vi "Teleop.vi"(10 "Match Info":T1={"Autonomous Elapsed Seconds"=0.0, "TeleOp Elapsed Seconds"=0.0, "Disabled Elapsed Seconds"=0.0, "Visited Autonomous"=FALSE, "Visited TeleOp"=FALSE, "Visited Disabled"=FALSE, "Autonomous Settings"={"Autonomous Style"=enum."Independent", "VI Refnum"=refnum}}, 11 "Call Context":T2) -> ()   [LabVIEW 2019]
doc: "This VI is called for each TeleOp packet received from the DS where the robot is not disabled. It is often used to read from the joysticks and update I/O or to update setpoints for timed control loops. It should complete and return within 20 milliseconds or it may miss DS packets."
uses:
  <vilib>/Rock Robotics/WPI/DriverStation/WPI_DriverStationDerivedRobotMode.ctl
  <vilib>/Rock Robotics/WPI/DriverStation/WPI_DriverStationMatch Info.ctl
  <vilib>/Rock Robotics/WPI/DriverStation/WPI_DriverStationRobotMode2.ctl
  <vilib>/Rock Robotics/WPI/Utilities/WPI_GetSetVariantRefNum.vi
  Robot Global Data.vi
  <vilib>/Rock Robotics/Network Tables/NT Write Number.vi
  <vilib>/Rock Robotics/Network Tables/NT Write Boolean.vi
  <vilib>/Rock Robotics/WPI/RobotDrive/WPI_RobotDriveArcadeDrive_Standard(NoSaturation).vi
  <vilib>/Rock Robotics/Network Tables/NT Write Numeric Array.vi
  <vilib>/Analysis/NI_AALPro.lvlib
  <vilib>/Rock Robotics/WPI/ThirdParty/REV Robotics/SPARK MAX/Typedef/Spark MAX Control Type.ctl
panel:
  in  "error in":errorcluster
  # "Click here to set min"
  # "Click here to set max"
  # "Click here to set min"
  # "Click here to set max"
  # "Click here to set min"
  # "Click here to set max"
  # "Click here to set min"
  # "Click here to set max"
  # "Click here to set min"
  # "Click here to set max"
  # "Click here to set min"
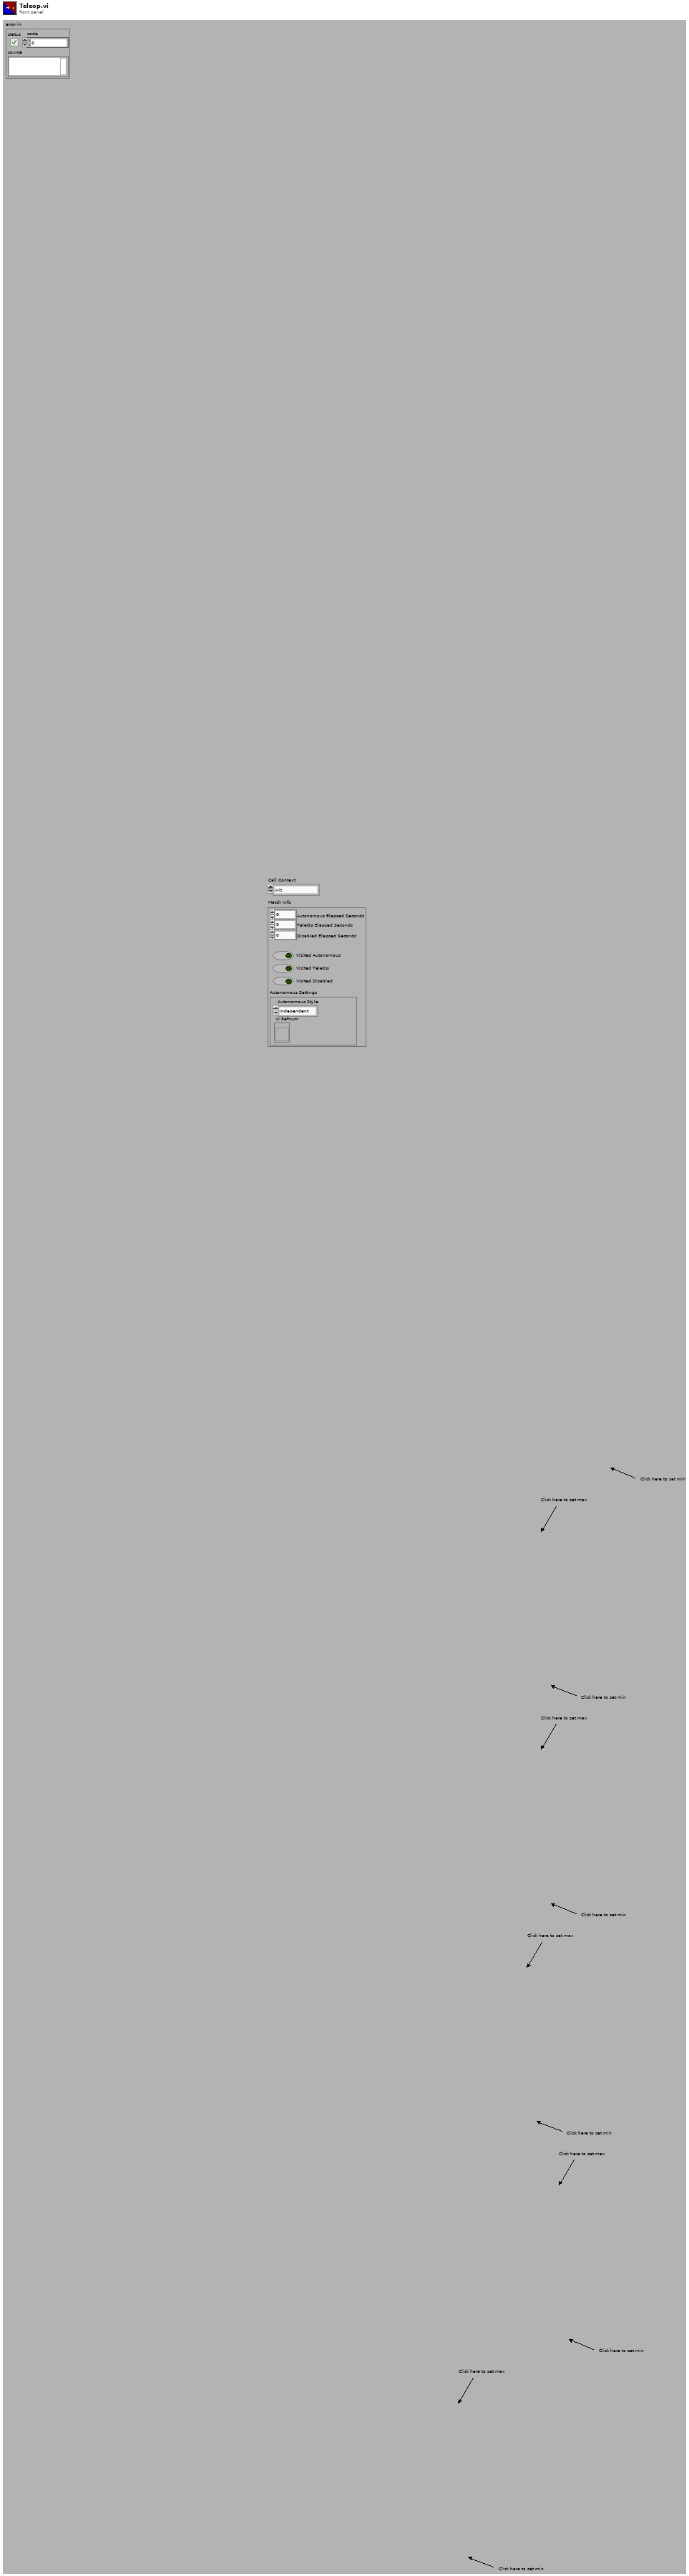
[diagram p1: front panel]
types:
  T1 = typedef "WPI_DriverStationMatch Info.ctl" = cluster{"Autonomous Elapsed Seconds":dbl, "TeleOp Elapsed Seconds":dbl, "Disabled Elapsed Seconds":dbl, "Visited Autonomous":bool, "Visited TeleOp":bool, "Visited Disabled":bool, "Autonomous Settings":cluster{"Autonomous Style":enum16{"Iterative", "Independent"}, "VI Refnum":refnum<vi>}}
  T2 = typedef "WPI_DriverStationDerivedRobotMode.ctl" = enum16{"Init", "Execute", "Stop"}
  T3 = typedef "WPI_MotorControlDeviceRef.ctl" = cluster{"DeviceStatus":errorcluster, "Type":T4, "PWM":cluster{"PWM Channel":T5, "DeadBand":T6}, "CAN":cluster{"Device Number":u8, "SetOutput VI Ref":variant, "GetOutput VI Ref":variant, "Enable VI Ref":variant, "Disable VI Ref":variant, "Data":variant}, "Invert":bool, "DIO PWM":cluster{"PWM \"Enable\" Channel":T5, "DIOChannel":T7, "PWM Rate":dbl}}
  T4 = typedef "WPI_MotorControlType.ctl" = enum16{"PWM", "CAN", "DIO PWM"}
  T5 = typedef "FPGA_DIOPWMChannel.ctl" = enum8{"PWM 0", "PWM 1", "PWM 2", "PWM 3", "PWM 4", "PWM 5", "PWM 6", "PWM 7", "PWM 8", "PWM 9", "PWM MXP 0", "PWM MXP 1", "PWM MXP 2", "PWM MXP 3", "PWM MXP 4", "PWM MXP 5", "PWM MXP 6", "PWM MXP 7", "PWM MXP 8", "PWM MXP 9", "Invalid"}
  T6 = typedef "WPI_PWMDeadband.ctl" = cluster{"Name":string, "maxPositivePwm":i32, "minPositivePwm":i32, "centerPwm":i32, "maxNegativePwm":i32, "minNegativePwm":i32, "angularRange":u16}
  T7 = typedef "FPGA_DIOChannel.ctl" = enum8{"DIO 0", "DIO 1", "DIO 2", "DIO 3", "DIO 4", "DIO 5", "DIO 6", "DIO 7", "DIO 8", "DIO 9", "DIO MXP 0", "DIO MXP 1", "DIO MXP 2", "DIO MXP 3", "DIO MXP 4", "DIO MXP 5", "DIO MXP 6", "DIO MXP 7", "DIO MXP 8", "DIO MXP 9", "DIO MXP 10", "DIO MXP 11", "DIO MXP 12", "DIO MXP 13", "DIO MXP 14", "DIO MXP 15", "SPI Port CS1", "SPI Port CS2", "SPI Port CS3", "SPI Port MISO", "SPI Port MOSI", "Invalid"}
  T8 = typedef "WPI_RobotDriveDevRef.ctl" = cluster{"DevStatus":errorcluster, "Motors[]":T3[], "Square Inputs":bool, "Max Output":dbl}
  T9 = typedef "WPI_ServoDeviceRef.ctl" = cluster{"DeviceStatus":errorcluster, "PWM Channel":T5, "DeadBand":T6}
  T10 = typedef "WPI_JoystickDevRef.ctl" = cluster{"Device":T11}
  T11 = typedef "WPI_JoystickDeviceEnum.ctl" = enum16{"USB 0", "USB 1", "USB 2", "USB 3", "USB 4", "USB 5"}
  T12 = typedef "Spark MAX Control Type.ctl" = enum16{"Percent VBus", "Voltage", "Velocity", "Position", "Smart Motion", "Current", "Smart Velocity"}
  T13 = typedef "WPI_DriverStationRobotMode2.ctl" = enum16{"Autonomous Disabled", "Autonomous Enabled", "Teleop Disabled", "Teleop Enabled", "Disconnected", "Finish", "Test Disabled", "Test Enabled", "Emergency Stopped"}
  T14 = cluster{"P Gain":dbl, "I Gain":dbl, "D Gain":dbl, "F Gain":dbl, "I Zone":dbl, "Min Output":dbl, "Max Output":dbl}
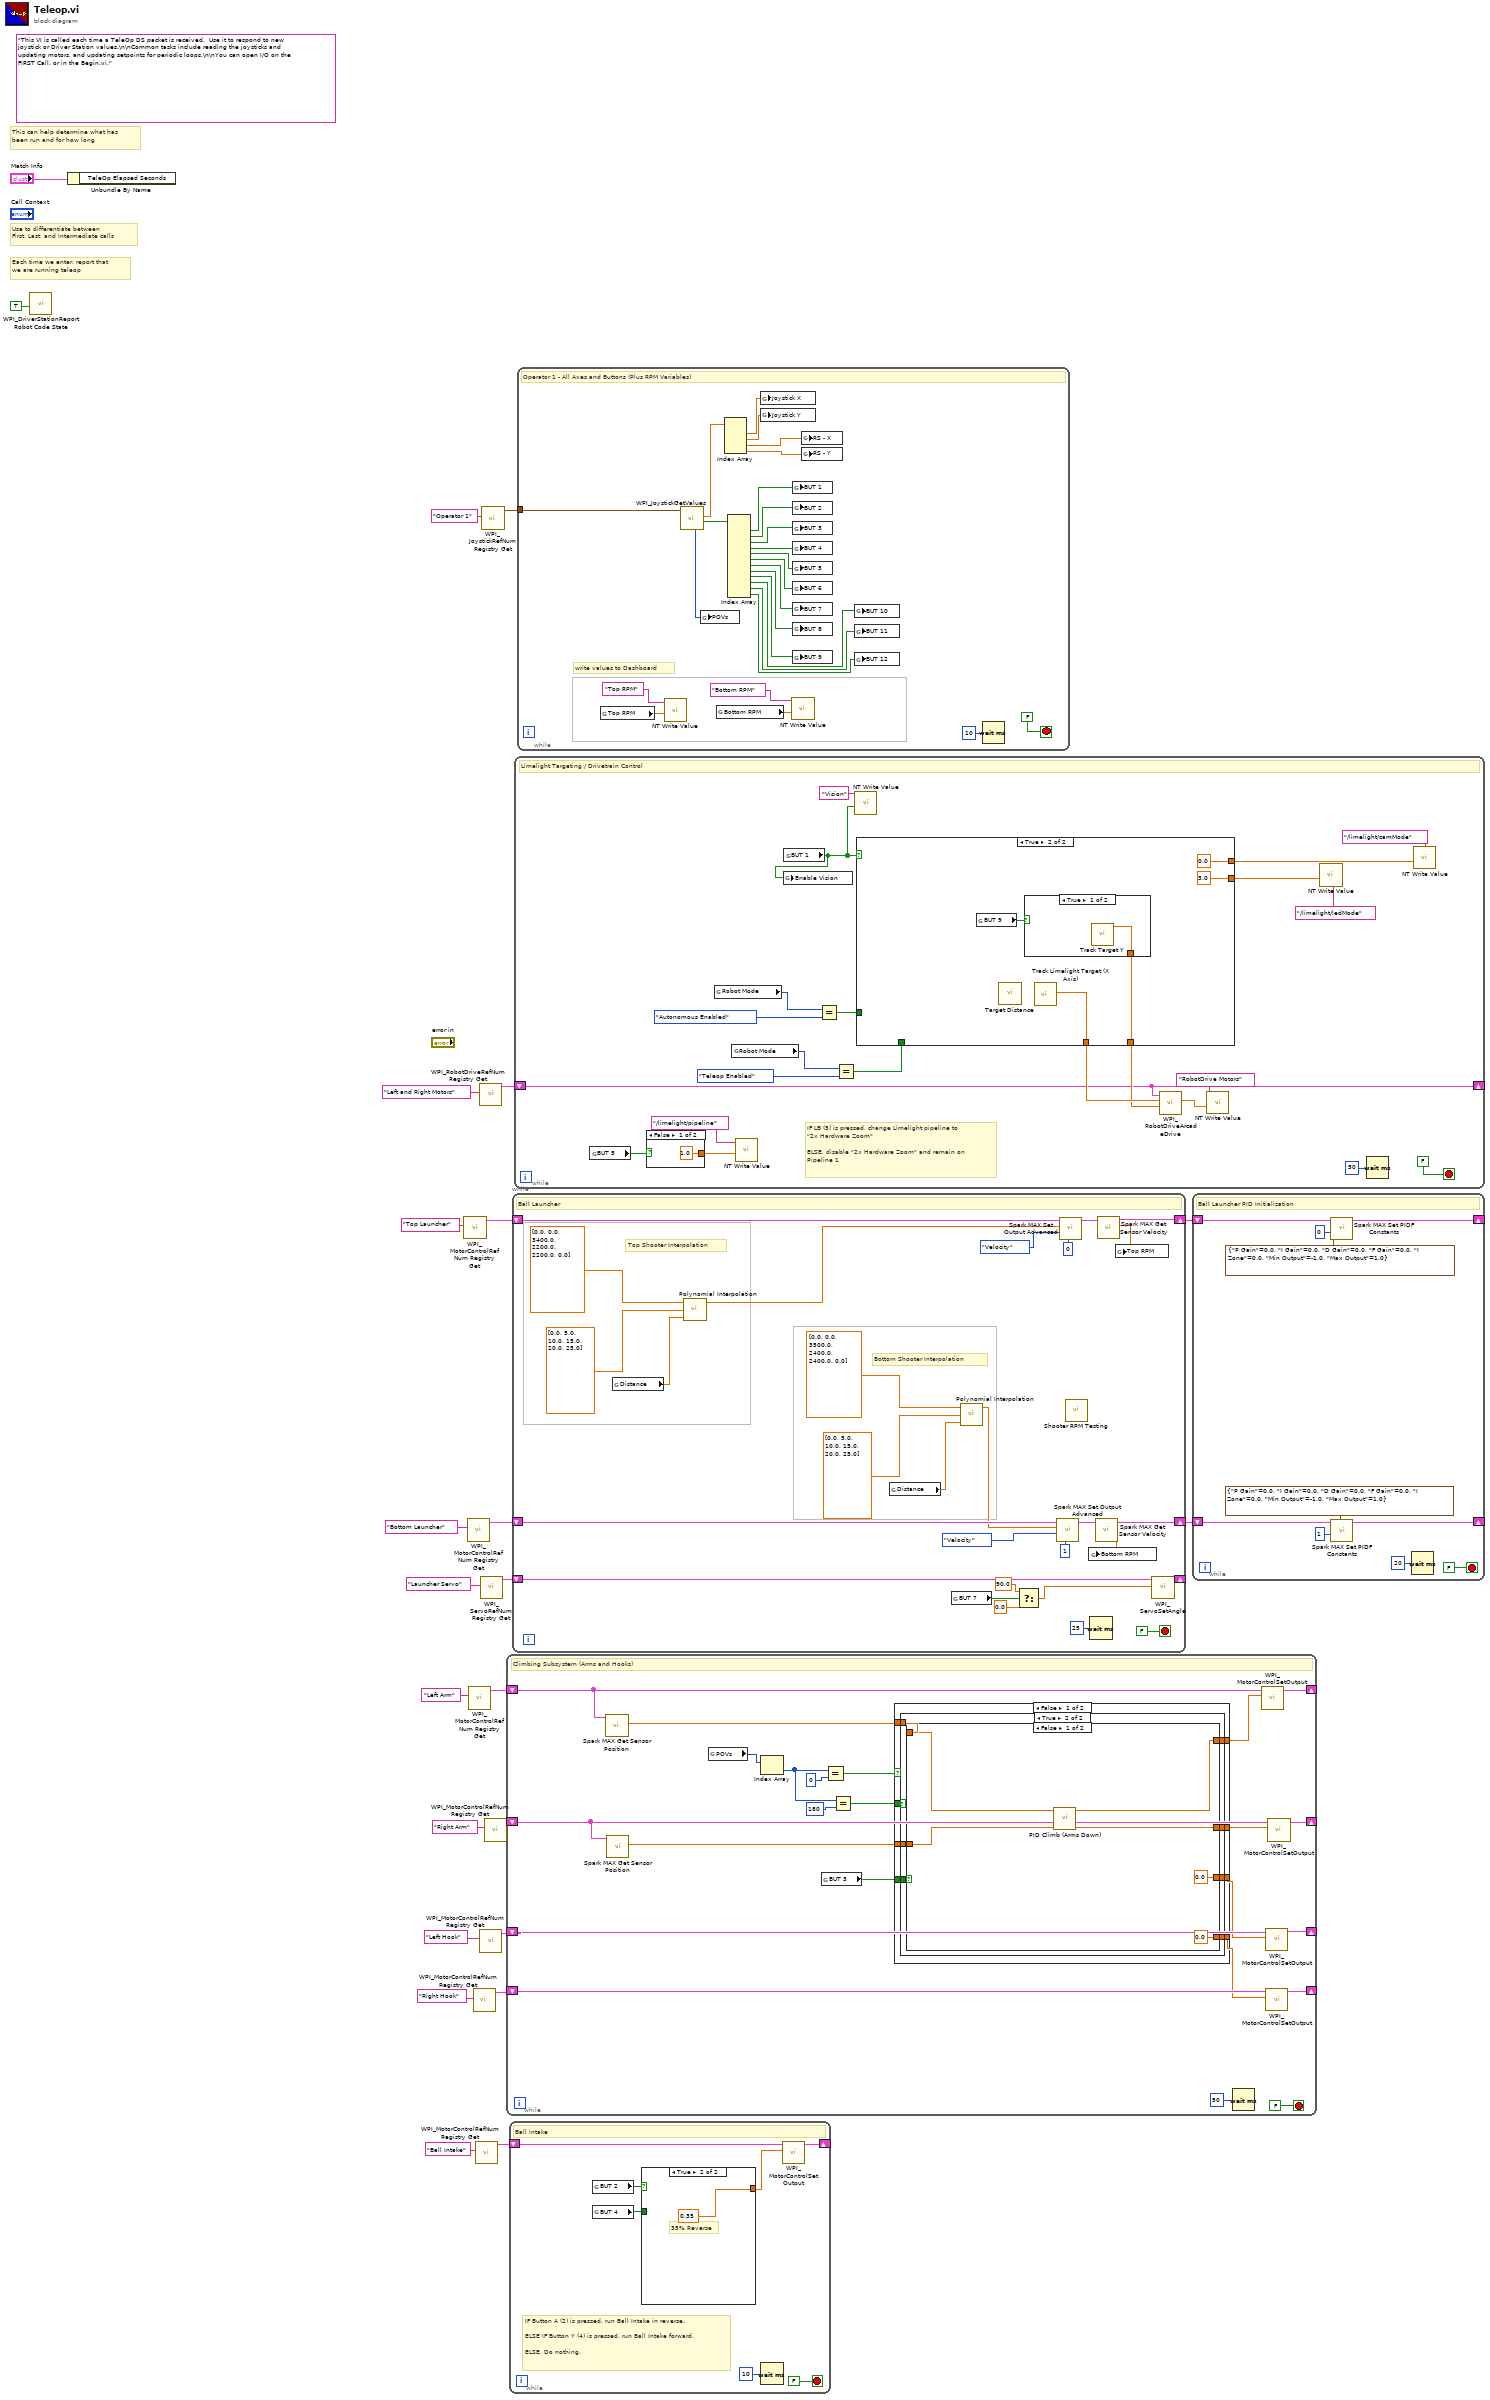
[diagram p0: block diagram]
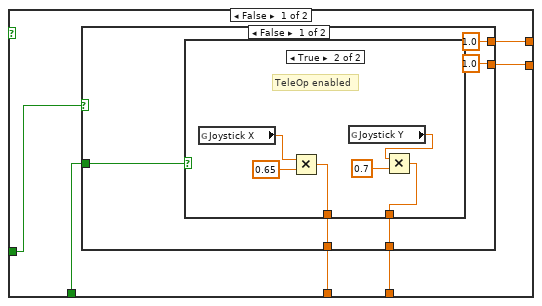
[diagram p2: hidden frame]
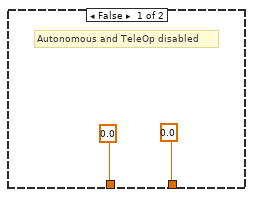
[diagram p3: hidden frame]
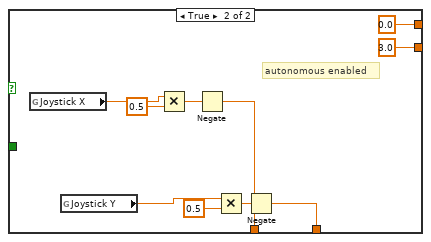
[diagram p4: hidden frame]
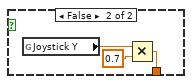
[diagram p5: hidden frame]
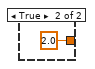
[diagram p6: hidden frame]
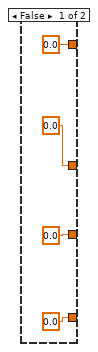
[diagram p7: hidden frame]
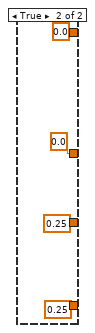
[diagram p8: hidden frame]
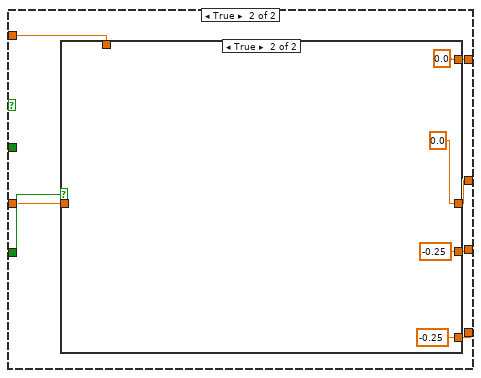
[diagram p9: hidden frame]
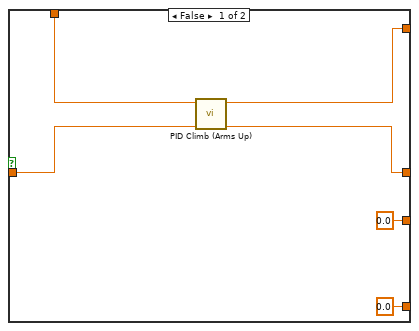
[diagram p10: hidden frame]
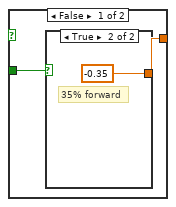
[diagram p11: hidden frame]
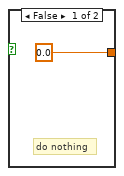
[diagram p12: hidden frame]
diagram:
  (unwired) "This VI is called each time a TeleOp DS packet is received.  Use it to respond to new joystick or Driver Station values.\n\nCommon tasks include reading the joysticks and updating motors, and updating setpoints for periodic loops.\n\nYou can open I/O on the FIRST Call, or in the Begin.vi."
  # "Each time we enter, report that\nwe are running teleop"
  # "Use to differentiate between\nFirst, Last, and Intermediate calls"
  # "This can help determine what has\nbeen run and for how long"
  n1 = call <vilib>:"WPI_DriverStationReport Robot Code State.vi"("TeleOp"=TRUE ("Autonomous")) -> ()  [unwired: 10 in, 1 out]
  n2 = Unbundle By Name("Match Info") -> ()  [unwired: 1 out]
  n3 = call <vilib>:"WPI_MotorControlRefNum Registry Get.vi"("refnum name"="Top Launcher") -> ("MotorControlDevRef"=w18:T3)  [unwired: 9 in, 1 out]
  n4 = call <vilib>:"WPI_MotorControlRefNum Registry Get.vi"("refnum name"="Bottom Launcher") -> ("MotorControlDevRef"=w20:T3)  [unwired: 9 in, 1 out]
  n5 = call <vilib>:"WPI_MotorControlRefNum Registry Get.vi"("refnum name"="Left Arm") -> ("MotorControlDevRef"=w12:T3)  [unwired: 9 in, 1 out]
  n6 = call <vilib>:"WPI_MotorControlRefNum Registry Get.vi"("refnum name"="Right Hook") -> ("MotorControlDevRef"=w9:T3)  [unwired: 9 in, 1 out]
  n7 = call <vilib>:"WPI_MotorControlRefNum Registry Get.vi"("refnum name"="Ball Intake") -> ("MotorControlDevRef"=w14:T3)  [unwired: 9 in, 1 out]
  n8 = call <vilib>:"WPI_RobotDriveRefNum Registry Get.vi"("refnum name"="Left and Right Motors") -> ("RobotDriveDevRef"=w3:T8)  [unwired: 1 in, 9 out]
  n9 = call <vilib>:"WPI_MotorControlRefNum Registry Get.vi"("refnum name"="Left Hook") -> ("MotorControlDevRef"=w10:T3)  [unwired: 9 in, 1 out]
  n10 = call <vilib>:"WPI_ServoRefNum Registry Get.vi"("refnum name"="Launcher Servo") -> ("ServoDeviceRef"=w16:T9)  [unwired: 9 in, 1 out]
  n11 = call <vilib>:"WPI_JoystickRefNum Registry Get.vi"("refnum name"="Operator 1") -> ("JoystickDevRef"=w6:T10)  [unwired: 1 in, 9 out]
  n12 = call <vilib>:"WPI_MotorControlRefNum Registry Get.vi"("refnum name"="Right Arm") -> ("MotorControlDevRef"=w11:T3)  [unwired: 9 in, 1 out]
  n13 = while {
    shift-right: [w38] -> _
    shift-left: w12 -> [w33]
    shift-right: [w39] -> _
    shift-left: w11 -> [w34]
    shift-right: [w44] -> _
    shift-left: w9 -> [w43]
    shift-right: [w45] -> _
    shift-left: w10 -> [w42]
    stop <- FALSE stop-if-true
    # "Climbing Subsystem (Arms and Hooks)"
    n14 = call <vilib>:"Spark MAX Get Sensor Position.vi"("MotorControlDevRef in"=w33) -> ("Sensor Position"=w32:dbl)  [unwired: 7 in, 3 out]
    n15 = call <vilib>:"Spark MAX Get Sensor Position.vi"("MotorControlDevRef in"=w34) -> ("Sensor Position"=w35:dbl)  [unwired: 7 in, 3 out]
    n16 = global read "Robot Global Data.vi" "POVs"() -> (w31:i16[])
    n17 = Index Array(array=w31) -> (element=w25:i16)  [unwired: 1 in]
    n18 = global read "Robot Global Data.vi" "BUT 3"() -> (w26:bool)
    n19 = Equal?(x=w25, y=i16 0) -> (x = y?=w28:bool)
    n20 = Equal?(x=w25, y=i16 180) -> (x = y?=w27:bool)
    n21 = case shown="False" w28 {
      tunnel: [w55 w80] -> w40
      tunnel: [w54 w79] -> w41
      tunnel: [w53 w81] -> w36
      tunnel: [w52 w82] -> w37
      tunnel: w27 -> [w51 _]
      tunnel: w26 -> [w50 w83]
      tunnel: w35 -> [w49 w78]
      tunnel: w32 -> [w48 w77]
      frame False {
        n22 = case shown="True" w51 {
          tunnel: [0.0 ("Output") w66] -> w55
          tunnel: [0.0 ("Output") w65] -> w54
          tunnel: [0.0 w64] -> w53
          tunnel: [0.0 w63] -> w52
          tunnel: w50 -> [_ w62]
          tunnel: w49 -> [_ w61]
          tunnel: w48 -> [_ w60]
          frame False {
          }
          frame True {
            n23 = case shown="False" w62 {
              tunnel: [0.0 ("Output") 0.25 ("Output")] -> w66
              tunnel: [0.0 ("Output") 0.25 ("Output")] -> w65
              tunnel: [w67 0.0] -> w64
              tunnel: [w69 0.0] -> w63
              tunnel: w61 -> [w68 _]
              tunnel: w60 -> [w70 _]
              frame False {
                n24 = call "PID Climb (Arms Down).vi"("R Sensor Position"=w68, "L Sensor Position"=w70) -> ("R Motor Output"=w67:dbl, "L Motor Output"=w69:dbl)  [unwired: 8 in]
              }
              frame True {
              }
            }
          }
        }
      }
      frame True {
        n25 = case shown="True" w83 {
          tunnel: [w85 0.0] -> w82
          tunnel: [w84 0.0] -> w81
          tunnel: [0.0 ("Output") -0.25 ("Output")] -> w80
          tunnel: [0.0 ("Output") -0.25 ("Output")] -> w79
          tunnel: w78 -> [w87 _]
          tunnel: w77 -> [w86 _]
          frame False {
            n26 = call "PID Climb (Arms Up).vi"("R Sensor Position"=w87, "L Sensor Position"=w86) -> ("R Motor Output"=w84:dbl, "L Motor Output"=w85:dbl)  [unwired: 8 in]
          }
          frame True {
          }
        }
      }
    }
    n27 = Wait (ms)(milliseconds to wait=u32 50) -> ()  [unwired: 1 out]
    n28 = call <vilib>:"WPI_MotorControlSetOutput.vi"("Output"=w37, "MotorControlDevRef"=w33) -> ("MotorControlDevRef"=w38:T3)  [unwired: 7 in, 2 out]
    n29 = call <vilib>:"WPI_MotorControlSetOutput.vi"("Output"=w40, "MotorControlDevRef"=w42) -> ("MotorControlDevRef"=w45:T3)  [unwired: 7 in, 2 out]
    n30 = call <vilib>:"WPI_MotorControlSetOutput.vi"("Output"=w41, "MotorControlDevRef"=w43) -> ("MotorControlDevRef"=w44:T3)  [unwired: 7 in, 2 out]
    n31 = call <vilib>:"WPI_MotorControlSetOutput.vi"("Output"=w36, "MotorControlDevRef"=w34) -> ("MotorControlDevRef"=w39:T3)  [unwired: 7 in, 2 out]
  }
  n32 = while {
    shift-right: [w97] -> _
    shift-left: w14 -> [w98]
    stop <- FALSE stop-if-true
    # "IF Button A (2) is pressed, run Ball Intake in reverse. \n\nELSE IF Button Y (4) is pressed, run Ball Intake forward.\n\nELSE, Do nothing."
    # "Ball Intake"
    n33 = global read "Robot Global Data.vi" "BUT 2"() -> (w95:bool)
    n34 = global read "Robot Global Data.vi" "BUT 4"() -> (w96:bool)
    n35 = case shown="True" w95 {
      tunnel: [w102 0.35 ("Output")] -> w94
      tunnel: w96 -> [w101 _]
      frame False {
        n36 = case shown="True" w101 {
          tunnel: [0.0 ("Output") -0.35 ("Output")] -> w102
          frame False {
            # "do nothing"
          }
          frame True {
            # "35% forward"
          }
        }
      }
      frame True {
        # "35% Reverse"
      }
    }
    n37 = Wait (ms)(milliseconds to wait=u32 10) -> ()  [unwired: 1 out]
    n38 = call <vilib>:"WPI_MotorControlSetOutput.vi"("Output"=w94, "MotorControlDevRef"=w98) -> ("MotorControlDevRef"=w97:T3)  [unwired: 7 in, 2 out]
  }
  n39 = while {
    shift-right: [w128] -> w1
    shift-left: w20 -> [w118]
    shift-right: [w126] -> w2
    shift-left: w18 -> [w127]
    shift-right: [w125] -> _
    shift-left: w16 -> [w120]
    stop <- FALSE stop-if-true
    # "Bottom Shooter Interpolation"
    # "Top Shooter Interpolation"
    # "Ball Launcher"
    n40 = global read "Robot Global Data.vi" "Distance"() -> (w115:dbl)
    n41 = call <vilib>:"Polynomial Interpolation.vi"("x value"=w115, "X"=dbl[] [0.0, 5.0, 10.0, 15.0, 20.0, 25.0], "Y"=dbl[] [0.0, 0.0, 3400.0, 2200.0, 2200.0, 0.0]) -> ("interpolation value"=w114:dbl)  [unwired: 2 out]
    n42 = global read "Robot Global Data.vi" "Distance"() -> (w109:dbl)
    n43 = global read "Robot Global Data.vi" "BUT 7"() -> (w124:bool)
    n44 = call <vilib>:"Polynomial Interpolation.vi"("x value"=w109, "X"=dbl[] [0.0, 5.0, 10.0, 15.0, 20.0, 25.0], "Y"=dbl[] [0.0, 0.0, 3500.0, 2400.0, 2400.0, 0.0]) -> ("interpolation value"=w108:dbl)  [unwired: 2 out]
    n45 = Select(t=90.0, s=w124, f=0.0) -> (s? t:f=w121:dbl)
    n46 = call <vilib>:"Spark MAX Set Output Advanced.vi"("PIDF Slot (0)"=1, "Control Mode"=Spark_MAX_Control_Type."Velocity", "Setpoint"=w108, "MotorControlDevRef"=w118) -> ("MotorControlDevRef"=w119:T3)  [unwired: 6 in, 1 out]
    n47 = call <vilib>:"Spark MAX Set Output Advanced.vi"("PIDF Slot (0)"=0, "Control Mode"=Spark_MAX_Control_Type."Velocity", "Setpoint"=w114, "MotorControlDevRef"=w127) -> ("MotorControlDevRef"=w133:T3)  [unwired: 6 in, 1 out]
    n48 = call "Shooter RPM Testing.vi"() -> ()  [unwired: 12 in]
    n49 = Wait (ms)(milliseconds to wait=u32 25) -> ()  [unwired: 1 out]
    n50 = call <vilib>:"Spark MAX Get Sensor Velocity.vi"("MotorControlDevRef in"=w119) -> ("Sensor Velocity"=w132:dbl, "MotorControlDevRef out"=w128:T3)  [unwired: 7 in, 2 out]
    n51 = global write "Robot Global Data.vi" "Bottom RPM"(w132) -> ()
    n52 = call <vilib>:"Spark MAX Get Sensor Velocity.vi"("MotorControlDevRef in"=w133) -> ("Sensor Velocity"=w131:dbl, "MotorControlDevRef out"=w126:T3)  [unwired: 7 in, 2 out]
    n53 = global write "Robot Global Data.vi" "Top RPM"(w131) -> ()
    n54 = call <vilib>:"WPI_ServoSetAngle.vi"("Angle"=w121, "ServoDeviceRef"=w120) -> ("ServoDeviceRef"=w125:T9)  [unwired: 8 in, 1 out]
  }
  n55 = while {
    shift-right: [w136] -> _
    shift-left: w3 -> [w136]
    stop <- FALSE stop-if-true
    # "IF LB (5) is pressed, change Limelight pipeline to \n\"2x Hardware Zoom\"\n\nELSE, disable \"2x Hardware Zoom\" and remain on\nPipeline 1"
    # "Limelight Targeting / Drivetrain Control"
    n56 = global read "Robot Global Data.vi" "BUT 5"() -> (w139:bool)
    n57 = case shown="False" w139 {
      tunnel: [1.0 ("Numeric") 2.0 ("Numeric")] -> w152
      frame False {
      }
      frame True {
      }
    }
    n58 = global read "Robot Global Data.vi" "Robot Mode"() -> (w147:T13)
    n59 = global read "Robot Global Data.vi" "Robot Mode"() -> (w143:T13)
    n60 = call-poly <vilib>:"NT Write Value.vi"("Numeric"=w152, "Name"="/limelight/pipeline") -> ()  [unwired: 9 in, 1 out]
    n61 = global read "Robot Global Data.vi" "BUT 1"() -> (w134:bool)
    n62 = global write "Robot Global Data.vi" "Enable Vision"(w134) -> ()
    n63 = Equal?(x=w147, y=WPI_DriverStationRobotMode2."Autonomous Enabled") -> (x = y?=w145:bool)
    n64 = Equal?(x=w143, y=WPI_DriverStationRobotMode2."Teleop Enabled") -> (x = y?=w142:bool)
    n65 = call-poly <vilib>:"NT Write Value.vi"("Boolean"=w134, "Name"="Vision") -> ()  [unwired: 9 in, 1 out]
    n66 = case shown="True" w134 {
      tunnel: [w158 0.0 ("Numeric")] -> w149
      tunnel: [w157 3.0 ("Numeric")] -> w148
      tunnel: [w161 w187] -> w140
      tunnel: w145 -> [w159 _]
      tunnel: w142 -> [w160 _]
      tunnel: [w156 w186] -> w141
      frame False {
        n67 = case shown="False" w159 {
          tunnel: [w165 w184] -> w161
          tunnel: [w166 w183] -> w156
          tunnel: w160 -> [w164 _]
          tunnel: [1.0 ("Numeric") 0.0 ("Numeric")] -> w158
          tunnel: [1.0 ("Numeric") 3.0 ("Numeric")] -> w157
          frame False {
            n68 = case shown="True" w164 {
              tunnel: [0.0 ("Joystick X") w172] -> w166
              tunnel: [0.0 ("Joystick Y") w169] -> w165
              frame False {
                # "Autonomous and TeleOp disabled"
              }
              frame True {
                # "TeleOp enabled"
                n69 = global read "Robot Global Data.vi" "Joystick X"() -> (w174:dbl)
                n70 = Multiply(x=w174, y=0.65) -> (x*y=w172:dbl)
                n71 = global read "Robot Global Data.vi" "Joystick Y"() -> (w171:dbl)
                n72 = Multiply(x=w171, y=0.7) -> (x*y=w169:dbl)
              }
            }
          }
          frame True {
            # "autonomous enabled"
            n73 = global read "Robot Global Data.vi" "Joystick X"() -> (w179:dbl)
            n74 = global read "Robot Global Data.vi" "Joystick Y"() -> (w175:dbl)
            n75 = Multiply(x=w179, y=0.5) -> (x*y=w180:dbl)
            n76 = Negate(x=w180) -> (-x=w183:dbl)
            n77 = Multiply(x=w175, y=0.5) -> (x*y=w176:dbl)
            n78 = Negate(x=w176) -> (-x=w184:dbl)
          }
        }
      }
      frame True {
        n79 = global read "Robot Global Data.vi" "BUT 9"() -> (w185:bool)
        n80 = call "Target Distance.vi"() -> ()  [unwired: 12 in]
        n81 = case shown="True" w185 {
          tunnel: [w190 w193] -> w187
          frame True {
            n82 = call "Track Target Y.vi"() -> ("Joystick Y"=w190:dbl)  [unwired: 11 in]
          }
          frame False {
            n83 = global read "Robot Global Data.vi" "Joystick Y"() -> (w192:dbl)
            n84 = Multiply(x=w192, y=0.7) -> (x*y=w193:dbl)
          }
        }
        n85 = call "Track Limelight Target (X Axis).vi"() -> ("Joystick X"=w186:dbl)  [unwired: 11 in]
      }
    }
    n86 = call-poly <vilib>:"WPI_RobotDriveArcadeDrive.vi"("Y axis value"=w140, "X axis value"=w141, "RobotDriveDevRef"=w136) -> ("Motor Values"=w137:dbl[])  [unwired: 6 in, 2 out]
    n87 = call-poly <vilib>:"NT Write Value.vi"("Numeric Array"=w137, "Name"="RobotDrive Motors") -> ()  [unwired: 9 in, 1 out]
    n88 = call-poly <vilib>:"NT Write Value.vi"("Numeric"=w148, "Name"="/limelight/ledMode" ("LED Mode")) -> ()  [unwired: 9 in, 1 out]
    n89 = Wait (ms)(milliseconds to wait=u32 50) -> ()  [unwired: 1 out]
    n90 = call-poly <vilib>:"NT Write Value.vi"("Numeric"=w149, "Name"="/limelight/camMode" ("Camera Mode")) -> ()  [unwired: 9 in, 1 out]
  }
  n91 = while {
    tunnel: w6 -> [w198]
    stop <- FALSE stop-if-true
    # "write values to Dashboard"
    # "Operator 1 - All Axes and Buttons (Plus RPM Variables)"
    n92 = global read "Robot Global Data.vi" "Top RPM"() -> (w203:dbl)
    n93 = call-poly <vilib>:"NT Write Value.vi"("Numeric"=w203, "Name"="Top RPM") -> ()  [unwired: 9 in, 1 out]
    n94 = call <vilib>:"WPI_JoystickGetValues.vi"("JoystickDevRef"=w198) -> ("Buttons"=w220:bool[], "Axes"=w207:dbl[], "POVs"=w199:i16[])  [unwired: 6 in, 2 out]
    n95 = global write "Robot Global Data.vi" "POVs"(w199) -> ()
    n96 = global read "Robot Global Data.vi" "Bottom RPM"() -> (w201:dbl)
    n97 = Index Array(array=w207) -> (element #1=w197:dbl, element #2=w196:dbl, element #3=w200:dbl, element #4=w206:dbl)  [unwired: 4 in]
    n98 = Index Array(array=w220) -> (element #1=w219:bool, element #2=w218:bool, element #3=w217:bool, element #4=w216:bool, element #5=w215:bool, element #6=w214:bool, element #7=w213:bool, element #8=w212:bool, element #9=w211:bool, element #10=w210:bool, element #11=w209:bool, element #12=w208:bool)  [unwired: 12 in]
    n99 = global write "Robot Global Data.vi" "Joystick X"(w197) -> ()
    n100 = global write "Robot Global Data.vi" "Joystick Y"(w196) -> ()
    n101 = call-poly <vilib>:"NT Write Value.vi"("Numeric"=w201, "Name"="Bottom RPM") -> ()  [unwired: 9 in, 1 out]
    n102 = global write "Robot Global Data.vi" "BUT 1"(w219) -> ()
    n103 = global write "Robot Global Data.vi" "BUT 2"(w218) -> ()
    n104 = global write "Robot Global Data.vi" "BUT 3"(w217) -> ()
    n105 = global write "Robot Global Data.vi" "BUT 4"(w216) -> ()
    n106 = global write "Robot Global Data.vi" "BUT 5"(w215) -> ()
    n107 = global write "Robot Global Data.vi" "BUT 6"(w214) -> ()
    n108 = global write "Robot Global Data.vi" "BUT 7"(w213) -> ()
    n109 = global write "Robot Global Data.vi" "BUT 8"(w212) -> ()
    n110 = global write "Robot Global Data.vi" "BUT 9"(w211) -> ()
    n111 = global write "Robot Global Data.vi" "RS - X"(w200) -> ()
    n112 = global write "Robot Global Data.vi" "RS - Y"(w206) -> ()
    n113 = global write "Robot Global Data.vi" "BUT 10"(w210) -> ()
    n114 = global write "Robot Global Data.vi" "BUT 11"(w209) -> ()
    n115 = global write "Robot Global Data.vi" "BUT 12"(w208) -> ()
    n116 = Wait (ms)(milliseconds to wait=u32 10) -> ()  [unwired: 1 out]
  }
  n117 = while {
    shift-right: [w230] -> _
    shift-left: w2 -> [w231]
    shift-right: [w228] -> _
    shift-left: w1 -> [w229]
    stop <- FALSE stop-if-true
    # "Ball Launcher PID Initialization"
    n118 = call <vilib>:"Spark MAX Set PIDF Constants.vi"("PIDF Slot"=0, "PID Constants"=T14 {"P Gain"=0.0, "I Gain"=0.0, "D Gain"=0.0, "F Gain"=0.0, "I Zone"=0.0, "Min Output"=-1.0, "Max Output"=1.0}, "MotorControlDeviceRef"=w231) -> ("MotorControlDeviceRef"=w230:T3)  [unwired: 7 in, 1 out]
    n119 = call <vilib>:"Spark MAX Set PIDF Constants.vi"("PIDF Slot"=1, "PID Constants"=T14 {"P Gain"=0.0, "I Gain"=0.0, "D Gain"=0.0, "F Gain"=0.0, "I Zone"=0.0, "Min Output"=-1.0, "Max Output"=1.0}, "MotorControlDeviceRef"=w229) -> ("MotorControlDeviceRef"=w228:T3)  [unwired: 7 in, 1 out]
    n120 = Wait (ms)(milliseconds to wait=u32 20) -> ()  [unwired: 1 out]
  }
